vi "set channel.vi"(8 "error in":errorcluster, 10 "TBM channel in":refnum<class "TBM channel.lvclass">, 11 "SHM configuration in":refnum<class "Shared Memory configuration.lvclass">) -> (0 "error out":errorcluster, 3 "SHM configuration out":refnum<class "Shared Memory configuration.lvclass">)   [LabVIEW 2013, in "Shared Memory configuration.lvclass"]
doc: "This function is responsible for replacing a channel, by name in the configuration class."
uses:
  module/configuration/Shared Memory configuration.lvclass
  <vilib>/NI/Tag Bus Module Framework/channel/TBM channel.lvclass
  <vilib>/NI/Tag Bus/tag/tag descriptor.lvclass/tag descriptor.ctl
  module/configuration/Shared Memory configuration.lvclass/Shared Memory configuration.ctl
  <vilib>/NI/Tag Bus/tag/tag descriptor.lvclass
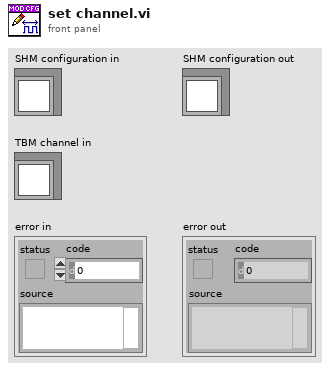
[diagram p1: front panel]
types:
  T1 = typedef "Shared Memory configuration.lvclass/Line.ctl" = cluster{"channel":refnum<class "TBM channel.lvclass">}
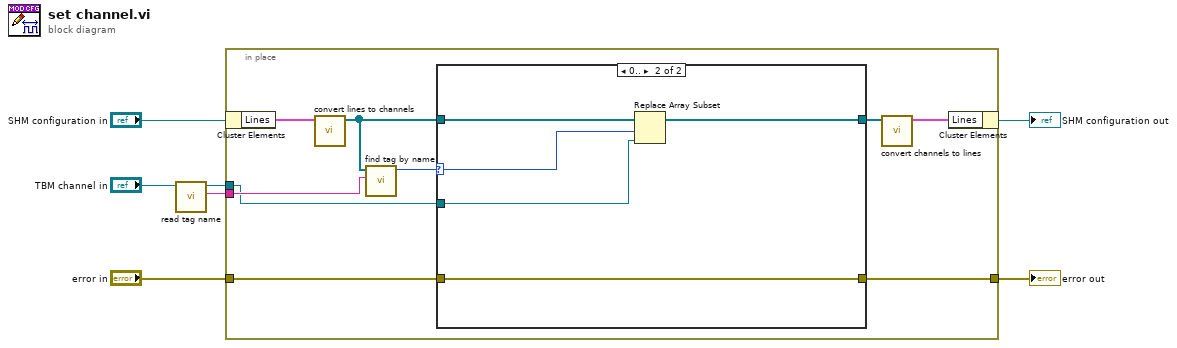
[diagram p0: block diagram]
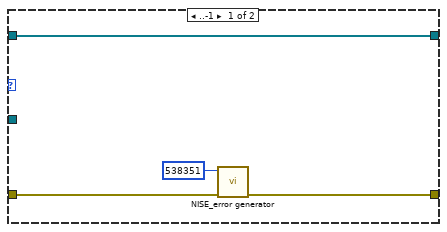
[diagram p2: hidden frame]
diagram:
  n1 = call <vilib>:"read tag name.vi"("system tag in"="TBM channel in") -> ("name"=w6:string, "system tag out"=w7:refnum<class "TBM channel.lvclass">)  [unwired: 8 in, 1 out]
  n2 = in-place {
    in-place-border: [w16] -> w4
    in-place-border: "error in" -> [w15]
    in-place-border: w7 -> [w13]
    in-place-border: w6 -> [w14]
    n3 = in-place-cluster #1("SHM configuration in") -> ("Lines"=w11:T1[])
    n4 = call "convert lines to channels.vi"("Lines in"=w11) -> ("channels out"=w10:refnum<class "TBM channel.lvclass">[])  [unwired: 9 in, 1 out]
    n5 = call <vilib>:"find tag by name.vi"("name"=w14, "tags in"=w10) -> ("index"=w12:i32)  [unwired: 9 in]
    n6 = case shown="0.." w12 {
      selector: w12 -> [_ w21]
      tunnel: w10 -> [w18 w24]
      tunnel: [w19 w25] -> w16
      tunnel: [w18 w23] -> w9
      tunnel: w15 -> [w17 w25]
      tunnel: w13 -> [_ w22]
      frame ..-1 {
        n7 = call <vilib>:"NISE_error generator.vi"("error in"=w17, "error code (0)"=538351) -> ("error out"=w19:errorcluster)  [unwired: 7 in]
      }
      frame 0.. {
        n8 = Replace Array Subset(array=w24, new element=w22, index=w21) -> (w23:refnum<class "TBM channel.lvclass">[])
      }
    }
    n9 = call "convert channels to lines.vi"("channels"=w9) -> ("Lines"=w8:T1[])  [unwired: 9 in, 1 out]
    n10 = in-place-cluster #1("Lines"=w8) -> (→"SHM configuration out":refnum<class "Shared Memory configuration.lvclass">)
  }
  "error out" <- w4
